vi "Epoch_Seconds Format String.vi"(7 "Delimiter (system)":T1, 10 "Unit (ms)":T2=enum."millisecond") -> (2 "format string":string)   [LabVIEW 2013]
uses:
  Seconds Units -- enum.ctl
  Locale -- enum.ctl
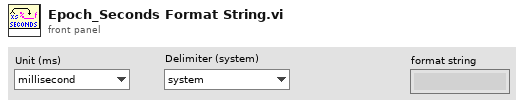
[diagram p1: front panel]
types:
  T1 = typedef "Locale -- enum.ctl" = enum16{"system", "Dot notation", "Comma notation", "custom"}
  T2 = typedef "Seconds Units -- enum.ctl" = enum16{"second", "millisecond", "microsecond", "nanosecond"}
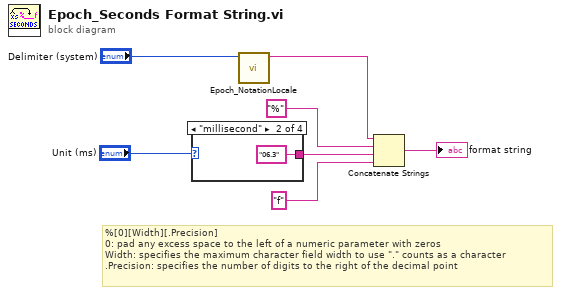
[diagram p0: block diagram]
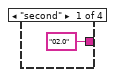
[diagram p2: hidden frame]
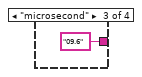
[diagram p3: hidden frame]
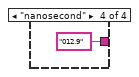
[diagram p4: hidden frame]
diagram:
  # "%[0][Width][.Precision]\n0: pad any excess space to the left of a numeric parameter with zeros\nWidth: specifies the maximum character field width to use \".\" counts as a character\n.Precision: specifies the number of digits to the right of the decimal point"
  n1 = case shown="\"millisecond\"" "Unit (ms)" {
    tunnel: ["02.0" "06.3" "09.6" "012.9"] -> w5
    frame "second" {
    }
    frame "millisecond" {
    }
    frame "microsecond" {
    }
    frame "nanosecond" {
    }
  }
  n2 = call "Epoch_NotationLocale.vi"("Delimiter (system)"="Delimiter (system)") -> ("delimiter format"=w1:string)  [unwired: 10 in]
  n3 = Concatenate Strings(w1, "%", w5, "f") -> (→"format string":string)
